vi "Configuration.vi"(8 "error in (no error)":errorcluster, 10 "RoiFilter":T1, 11 "Modeli in":refnum<class "Modeli.lvclass">) -> (0 "error out":errorcluster, 3 "Modeli out":refnum<class "Modeli.lvclass">)   [LabVIEW 2018, in "Modeli.lvlib" / "Modeli.lvclass"]
uses:
  Modeli.lvclass
  C:/AME Test Engineering/LabVIEW/PPLs/Sensor/Parent/Sensor.lvlibp/Sensor.lvclass
  Projects/PRJ-Quasar Listening/Quasar Listening/x64/Release/Quasar Listening.dll
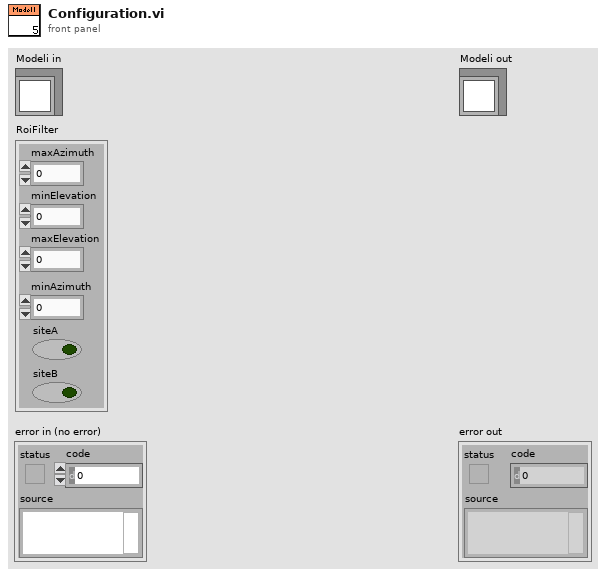
[diagram p1: front panel]
types:
  T1 = cluster{"minAzimuth":dbl, "maxAzimuth":dbl, "minElevation":dbl, "maxElevation":dbl, "siteA":bool, "siteB":bool}
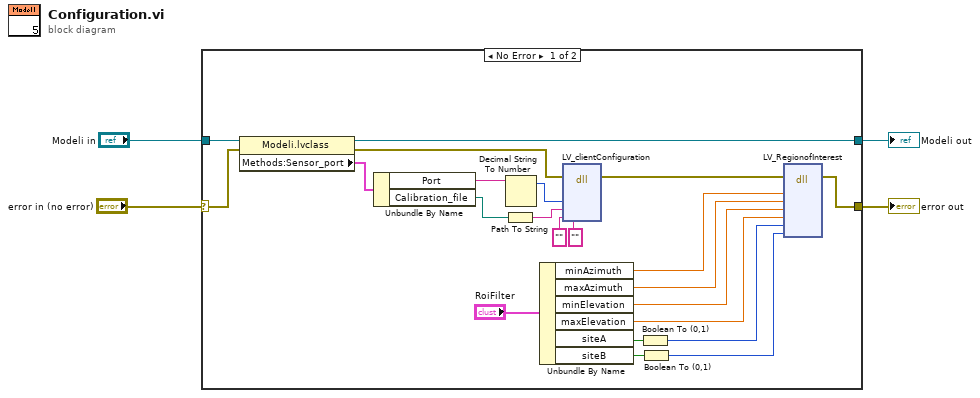
[diagram p0: block diagram]
diagram:
  n1 = case shown="No Error" "error in (no error)" {
    selector: "error in (no error)" -> [w18 w27]
    tunnel: "Modeli in" -> [w26 w28]
    tunnel: [w17 w27] -> w2
    tunnel: [w16 w28] -> w1
    frame No Error {
      n2 = property class="Modeli.lvclass"(reference=w26, error in=w18) -> (reference out=w16:refnum<class "Modeli.lvclass">, error out=w20:errorcluster, "Methods:Sensor_port"=w25:cluster{"Port":string, "Calibration_file":path})
      n3 = Unbundle By Name(w25) -> ("Port"=w23:string, "Calibration_file"=w22:path)
      n4 = Path To String(path=w22) -> (string=w21:string)
      n5 = Decimal String To Number(string=w23) -> (offset past number=w24:i32)  [unwired: 2 in, 1 out]
      n6 = Unbundle By Name("RoiFilter") -> ("minAzimuth"=w5:dbl, "maxAzimuth"=w6:dbl, "minElevation"=w7:dbl, "maxElevation"=w8:dbl, "siteA"=w12:bool, "siteB"=w11:bool)
      n7 = dll-call lib="C:/Projects/PRJ-Quasar Listening/Quasar Listening/x64/Release/Quasar Listening.dll" fn="LV_clientConfiguration"(error in=w20, "source_ip"="", "destination_port"=w24, "detector_calibration"=w21, "detector_configuration"="") -> (error out=w19:errorcluster)  [unwired: 7 in, 1 out]
      n8 = Boolean To (0,1)(Boolean=w12) -> (0, 1=w9:i16)
      n9 = Boolean To (0,1)(Boolean=w11) -> (0, 1=w10:i16)
      n10 = dll-call lib="C:/Projects/PRJ-Quasar Listening/Quasar Listening/x64/Release/Quasar Listening.dll" fn="LV_RegionofInterest"(error in=w19, "minAzimuth"=w5, "maxAzimuth"=w6, "minElevation"=w7, "maxElevation"=w8, "siteA"=w9, "siteB"=w10) -> (error out=w17:errorcluster)  [unwired: 9 in, 1 out]
    }
    frame Error {
    }
  }
  "error out" <- w2
  "Modeli out" <- w1
